vi "Meas Result Make Unc Bars to Graph.vi"(3 "independent":dbl[](array[numeric]), 4 "unc":dbl[](array[numeric]), 5 "mean":dbl[](array[numeric])) -> (0 "trace":cluster{dbl[], dbl[]}, 1 "unc out":dbl[](array[numeric]), 2 "independent out":dbl[](array[numeric]))   [LabVIEW 2020]
doc: "Simulates uncertainty bars to graph by inserting vertical element to vector of graph values."
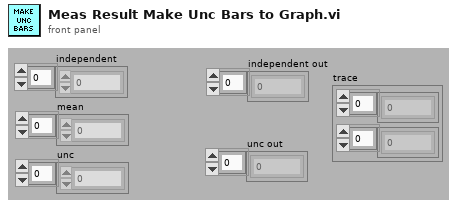
[diagram p1: front panel]
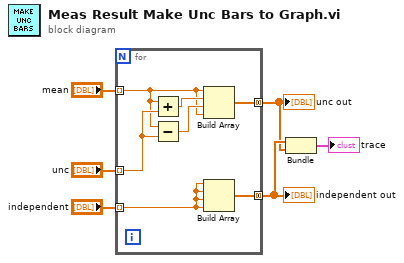
[diagram p0: block diagram]
diagram:
  n1 = for {
    tunnel: "mean" -> [w10] mode=indexing
    tunnel: "unc" -> [w12] mode=indexing
    tunnel: "independent" -> [w9] mode=indexing
    tunnel: [w8] -> w2 mode=concatenating
    tunnel: [w7] -> w3 mode=concatenating
    n2 = Add(x=w10, y=w12) -> (x+y=w13:dbl)
    n3 = Subtract(x=w10, y=w12) -> (x-y=w11:dbl)
    n4 = Build Array(w10, w13, w11, w10) -> (w8:dbl[])
    n5 = Build Array(w9, w9, w9, w9) -> (w7:dbl[])
  }
  "independent out" <- w3
  "unc out" <- w2
  n6 = Bundle(w3, w2) -> (→"trace":cluster{dbl[], dbl[]})  [unwired: 1 in]
